vi "Cruise Control.vi"() -> ()   [LabVIEW 2018]
uses:
  <vilib>/Simulation/Scripting/Companion Diagram/SimConfigNode/SimParams.ctl
  <vilib>/Simulation/Scripting/Companion Diagram/SimConfigNode/_simSolvers.ctl
  <vilib>/Simulation/Implementation/Shared/SIMSCR Execution Mode.ctl
  <vilib>/Platform/TimedLoop/XDataNode/timing_clust.ctl
  <vilib>/Platform/TimedLoop/XDataNode/nitl_modes.ctl
  <vilib>/Platform/TimedLoop/XDataNode/wakeup.ctl
  <vilib>/Simulation/Param Hierarchy/Typedefs/SIMPH Param Control Actions.ctl
  <vilib>/Quanser/Rapid Control Prototyping Toolkit/communications/basic/Basic Stream Receive Mode.ctl
  <vilib>/Quanser/Rapid Control Prototyping Toolkit/communications/basic/Basic Stream Send Mode.ctl
  <vilib>/Simulation/Implementation/Shared/NILVSim_FinalizeModel.vi
  <vilib>/Simulation/Implementation/Shared/NILVSim_FinishedLate.vi
  <vilib>/Simulation/Utility/Implementation/SIM Halt.vi
  <vilib>/Simulation/SignalArithmetic/Implementation/NILVSim Gain.llb/SIM Gain (scalar).vi
  <vilib>/Simulation/Utility/Implementation/NILVSim Memory.llb/NILVSim Memory (core).vi
  <vilib>/Simulation/Implementation/Shared/NILVSim_Manager.vi
  <vilib>/Simulation/Implementation/Shared/NILVSIM_BeginStep.vi
  <vilib>/Simulation/Implementation/Shared/NILVSim_ParamChanged.vi
  <vilib>/Utility/error.llb/Clear Errors.vi
  <vilib>/Simulation/Implementation/Shared/SIM Unbundle Sim Info.vi
  <vilib>/Simulation/Implementation/Shared/SIMSH Read Queue.vi
  <vilib>/Simulation/Implementation/Shared/NILVSim_Initialize.vi
  <vilib>/Simulation/Utility/Implementation/NILVSim Get Time and IsAcceptedStep.vi
  <vilib>/Simulation/Implementation/Shared/NILVSim_GetModelError.vi
  <vilib>/Simulation/Implementation/Shared/SIM Bundle Sim Info.vi
  <vilib>/Simulation/Scripting/Companion Diagram/SimConfigNode/SimDog.xnode
  SubVIs/Animate.vi
  SubVIs/Auto_Driver.vi
  SubVIs/Track_Model.vi
  SubVIs/Navigation_Sensors_G.vi
  <vilib>/Quanser/Rapid Control Prototyping Toolkit/communications/basic/_TypeSpecific/CL Comm Basic Stream Client (DBL).vi
  <vilib>/Quanser/Rapid Control Prototyping Toolkit/communications/basic/CL Comm Basic Stream Client.vi
  <vilib>/Quanser/Rapid Control Prototyping Toolkit/visualization/Visualization.lvclass
  <vilib>/Platform/TimedLoop/XDataNode/XDataNode.xnode
  <vilib>/Simulation/Implementation/XNodeFramework/SimXNode/SimX.xnode
  <vilib>/Platform/TimedLoop/XDataNode/XDNodeRunTimeDep.lvlib
  <vilib>/Simulation/Implementation/Shared/NI_SIM_Implementation.lvlib
panel:
  out "Speed Response":cluster{"output":dbl, "Desired_Speed":dbl}(graph)
  in  "Speed Ki":dbl=0.1
  in  "Speed Kp":dbl=0.01
  out "Speed (km/h)":dbl(knob)=139.07123712366658 scale=0.0..200.0
  out "Steering Angle (rad)":dbl(knob)=-0.001509315249644288 scale=2.0..-2.0
  in  "Stop":bool caption="START"
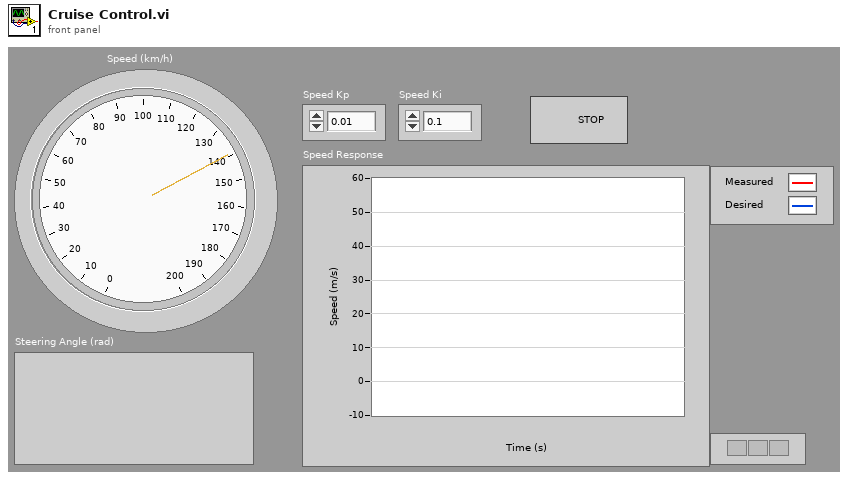
[diagram p1: front panel]
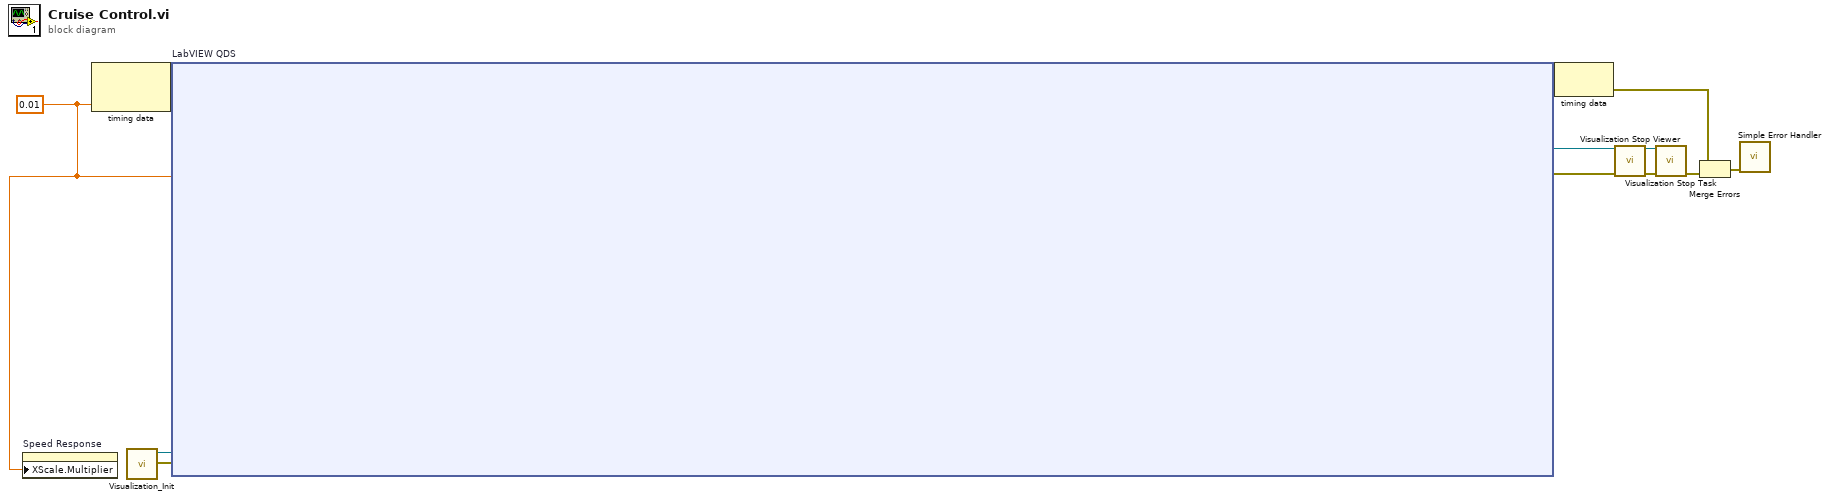
[diagram p0: block diagram]
diagram:
  w1 = 0.01 ("Step Size (s)")
  n1 = property on="Speed Response" class="WFChart (strict)"("XScale.Multiplier"=w1) -> ()  [unwired: 2 in, 2 out]
  n2 = node-c288(w1) -> (w12:variant)  [unwired: 1 in]
  n3 = call "Visualization_Init.vi"() -> ("error out"=w9:errorcluster, "visualization out"=w10:refnum<class "Visualization.lvclass">)  [unwired: 10 in]
  n4 = node-c254 "LabVIEW QDS"(w12, w10, w9, w1) -> (w11:variant, w3:errorcluster, w4:refnum<class "Visualization.lvclass">)
  n5 = node-c288(w11) -> (w7:errorcluster)
  n6 = call <vilib>:"Visualization Stop Viewer.vi"("visualization in"=w4, "error in (no error)"=w3) -> ("visualization out"=w6:refnum<class "Visualization.lvclass">, "error out"=w5:errorcluster)  [unwired: 12 in]
  n7 = call <vilib>:"Visualization Stop Task.vi"("visualization in"=w6, "error in (no error)"=w5) -> ("error out"=w2:errorcluster)  [unwired: 13 in]
  n8 = Merge Errors(w7, w2) -> (w8:errorcluster)
  n9 = call <vilib>:"Simple Error Handler.vi"("error in (no error)"=w8) -> ()  [unwired: 4 in, 5 out]
